vi "Get Message.vi"(0 "MLA":refnum<class "MLA.lvclass">, 1 "Loop":T1, 3 "Timeout (100mS)":i32=100, 5 "error in (no error)":errorcluster) -> (11 "Timeout?":bool, 13 "Raw Message":string, 14 "MLA":refnum<class "MLA.lvclass">, 15 "Message":string, 16 "Param 1":string, 17 "Param 2":string, 18 "Params":string[](array[string]), 19 "error out":errorcluster)   [LabVIEW 2023, in "MLA.lvclass"]
uses:
  MLA.lvclass
  controls/MLA Loops.ctl
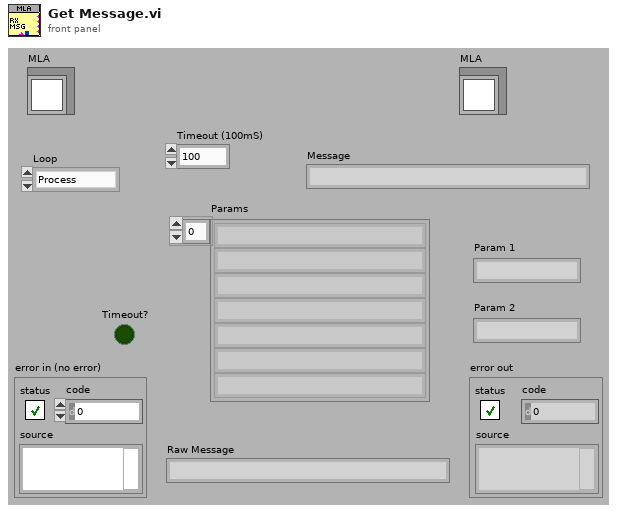
[diagram p1: front panel]
types:
  T1 = typedef "MLA Loops.ctl" = enum16{"Process", "REST", "WS"}
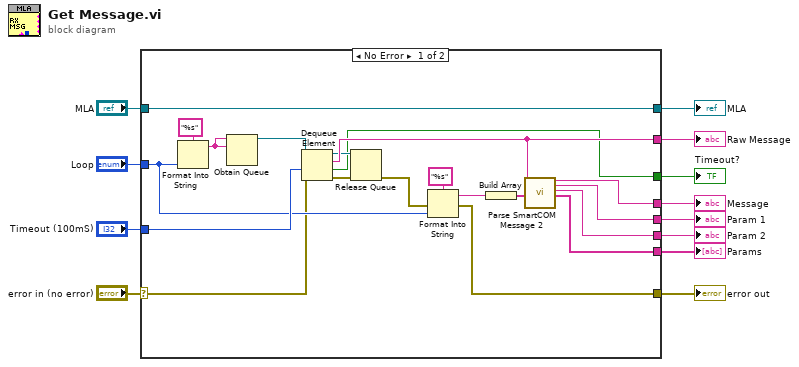
[diagram p0: block diagram]
diagram:
  n1 = case shown="No Error" "error in (no error)" {
    selector: "error in (no error)" -> [w18 w34]
    tunnel: [w23 w34] -> w11
    tunnel: [w17 w33] -> w9
    tunnel: "MLA" -> [w17 w33]
    tunnel: "Loop" -> [w20 _]
    tunnel: [w32 _] -> w7
    tunnel: [w31 _] -> w6
    tunnel: [w30 _] -> w5
    tunnel: [w29 _] -> w4
    tunnel: [w28 _] -> w3
    tunnel: "Timeout (100mS)" -> [w27 _]
    tunnel: [w13 _] -> w1
    frame No Error {
      n2 = Format Into String(format string="%s", w20) -> (resulting string=w21:string)  [unwired: 2 in, 1 out]
      n3 = Obtain Queue(name (unnamed)=w21, element data type=w21) -> (queue out=w19:refnum<queue>)  [unwired: 3 in, 2 out]
      n4 = Dequeue Element(queue=w19, timeout in ms (-1)=w27, error in (no error)=w18) -> (queue out=w16:refnum<queue>, element=w32:string, timed out?=w13:bool, error out=w15:errorcluster)
      n5 = Release Queue(queue=w16, error in (no error)=w15) -> (error out=w14:errorcluster)  [unwired: 1 in, 2 out]
      n6 = Format Into String(format string="%s", error in=w14, w20) -> (resulting string=w24:string, error out=w23:errorcluster)  [unwired: 1 in]
      n7 = Build Array(w24) -> (w26:string[])
      n8 = call "Parse SmartCOM Message 2.vi"("Message"=w32, "Names"=w26) -> ("Root Message"=w31:string, "Param 1"=w30:string, "Param 2"=w29:string, "All Params"=w28:string[])  [unwired: 9 in, 5 out]
    }
    frame Error {
    }
  }
  "error out" <- w11
  "MLA" <- w9
  "Param 1" <- w5
  "Message" <- w6
  "Param 2" <- w4
  "Params" <- w3
  "Raw Message" <- w7
  "Timeout?" <- w1
